vi "XNET System Property Node.vi"   [LabVIEW 2018]
uses:
  <resource>/objmgr/xnet.rc
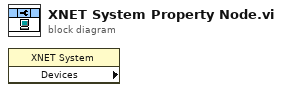
[diagram p0: block diagram]
diagram:
  n1 = property class="XNET System" props=["Devices"]() -> ()  [unwired: 2 in, 3 out]
